vi "FromJson.vi"(8 "error in (no error)":errorcluster, 10 "PersonnelJson":string) -> (0 "error out":errorcluster, 3 "Personnel out":refnum<class "Personnel.lvclass">)   [LabVIEW 2015, in "Personnel.lvclass"]
uses:
  Personnel.lvclass
  JsonCluster.ctl
  Personnel.lvclass/Personnel.ctl
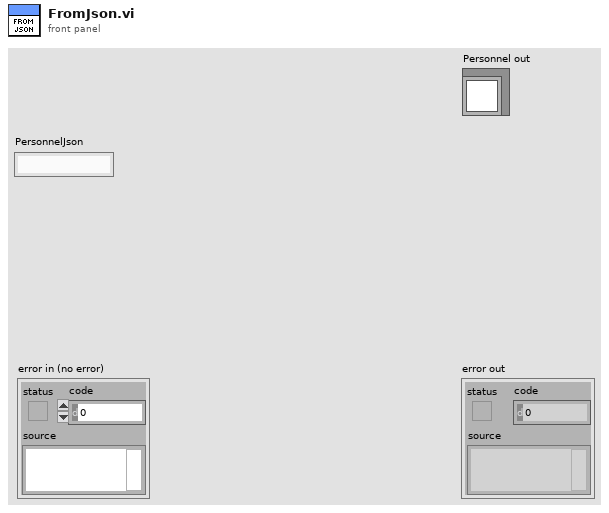
[diagram p1: front panel]
types:
  T1 = typedef "Personnel.lvclass/JsonCluster.ctl" = cluster{"Name":string, "Role":i32, "PUID":string, "Requests":string[]}
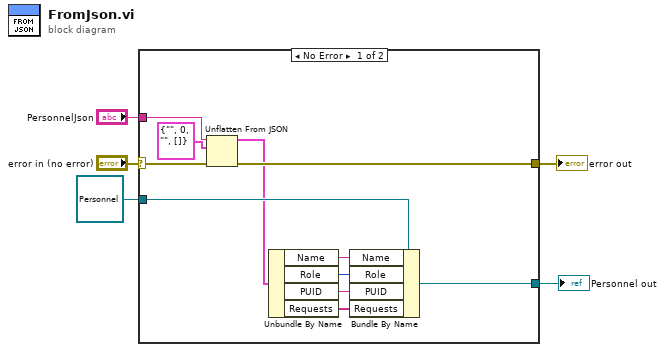
[diagram p0: block diagram]
diagram:
  n1 = case shown="No Error" "error in (no error)" {
    selector: "error in (no error)" -> [w12 w17]
    tunnel: [w11 w17] -> w4
    tunnel: [w8 w18] -> w2
    tunnel: refnum<class "Personnel.lvclass"> refnum ("Personnel in") -> [w9 w18]
    tunnel: "PersonnelJson" -> [w10 _]
    frame No Error {
      n2 = Unflatten From JSON(JSON string=w10, type and defaults=T1 {"Name"="", "Role"=0, "PUID"="", "Requests"=[]} ("Personal Json"), error in (no error)=w12) -> (value=w6:T1, error out=w11:errorcluster)  [unwired: 4 in]
      n3 = Unbundle By Name(w6) -> ("Name"=w16:string, "Role"=w15:i32, "PUID"=w14:string, "Requests"=w13:string[])
      n4 = Bundle By Name(cluster=w9, "Name"=w16, "Role"=w15, "PUID"=w14, "Requests"=w13) -> (w8:refnum<class "Personnel.lvclass">)
    }
    frame Error {
      # "Wire the error cluster across even in the \"No Error\"\ncase so that warnings get propagated."
    }
  }
  "error out" <- w4
  "Personnel out" <- w2
